vi "cmdLineParser.vi"(8 "error in (no error)":errorcluster, 11 "cmdLineArgs":string[](array[string])) -> (0 "error out":errorcluster, 1 "filesExist":bool, 2 "pathLvlibDir":path, 3 "pathIdl":path)   [LabVIEW 2018]
doc: "Command line parser to get the path of IDL and SAL LabVIEW vi."
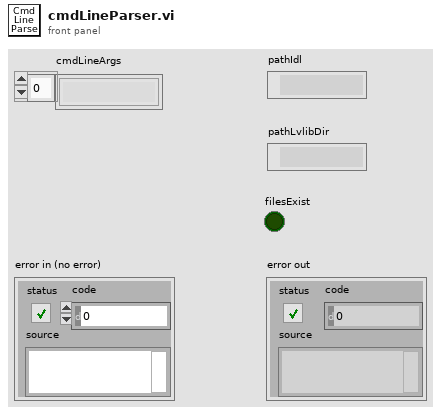
[diagram p1: front panel]
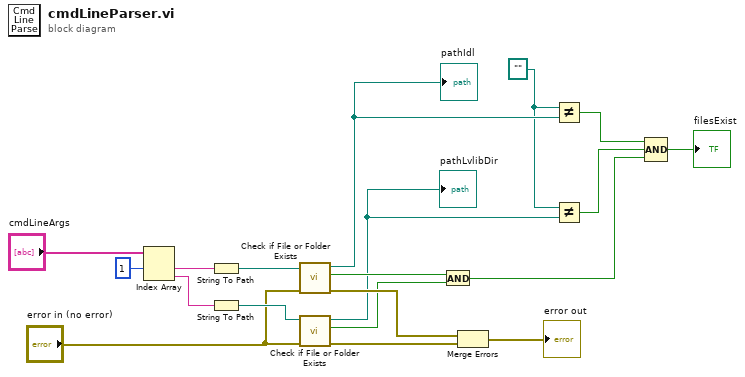
[diagram p0: block diagram]
diagram:
  w8 = path ""
  n1 = Index Array(array="cmdLineArgs", index #1=1 ("index")) -> (element #1=w18:string, element #2=w17:string)  [unwired: 1 in]
  n2 = String To Path(string=w18) -> (path=w16:path)
  n3 = String To Path(string=w17) -> (path=w15:path)
  n4 = call <vilib>:"Check if File or Folder Exists.vi"("error in (no error)"="error in (no error)", "path"=w16) -> ("error out"=w14:errorcluster, "file or folder exists?"=w11:bool, "dup path"=w9:path)  [unwired: 7 in]
  "pathIdl" <- w9
  n5 = call <vilib>:"Check if File or Folder Exists.vi"("error in (no error)"="error in (no error)", "path"=w15) -> ("error out"=w13:errorcluster, "file or folder exists?"=w10:bool, "dup path"=w7:path)  [unwired: 7 in]
  "pathLvlibDir" <- w7
  n6 = And(x=w11, y=w10) -> (x .and. y?=w4:bool)
  n7 = Merge Errors(w14, w13) -> (→"error out":errorcluster)
  n8 = Not Equal?(x=w8, y=w9) -> (x != y?=w6:bool)
  n9 = Not Equal?(x=w8, y=w7) -> (x != y?=w5:bool)
  n10 = Compound Arithmetic op=AND(w6, w5, w4) -> (→"filesExist":bool)
